vi "Binary_Gray.vi"() -> ()   [LabVIEW 2024]
panel:
  out "g0":bool
  in  "b0":bool
  out "g1":bool
  in  "b1":bool
  out "g3":bool
  in  "b2":bool
  out "g2":bool
  in  "b3":bool
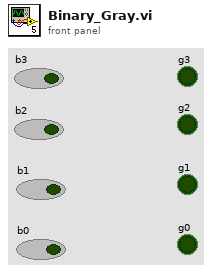
[diagram p1: front panel]
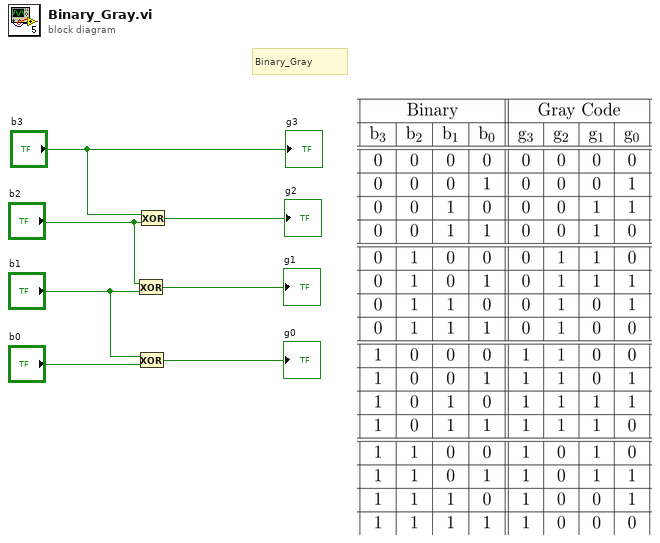
[diagram p0: block diagram]
diagram:
  # "Binary_Gray"
  n1 = Exclusive Or(1:"b1", 2:"b2") -> (0:→"g1":bool)
  n2 = Exclusive Or(1:"b0", 2:"b1") -> (0:→"g0":bool)
  n3 = Exclusive Or(1:"b2", 2:"b3") -> (0:→"g2":bool)
  "g3" <- "b3"
